vi "WFS Calc Spot To Reference Deviations.vi"(8 "error in (no error)":errorcluster {"code" format="%.0x"}, 10 "Cancel Wavefront Tilt (No)":i32(ring) items=["No", "Yes"], 11 "instrument handle":refnum<visa-resource-name>) -> (0 "error out":errorcluster {"code" format="%.0x"}, 3 "instrument handle out":refnum<visa-resource-name>)   [LabVIEW 2020]
doc: "This VI calculates reference positions and deviations for all spots depending on the setting ref_idx(internal/user) set by VI SetWavefrontReference.\nWhen option CancelWavefrontTilt is enabled the mean deviation in X and Y direction, which is measured within the pupil, is subtracted from the deviation data arrays.\n\nReference positions can be retrieved using VI GetSpotReferencePositions and calculated deviations by VI GetSpotDeviations."
uses:
  WFS_32.dll
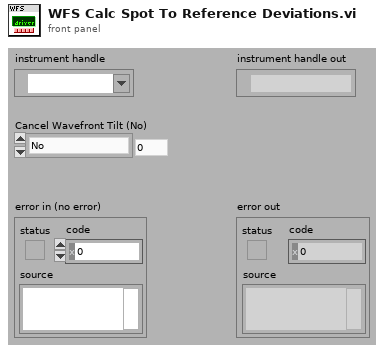
[diagram p1: front panel]
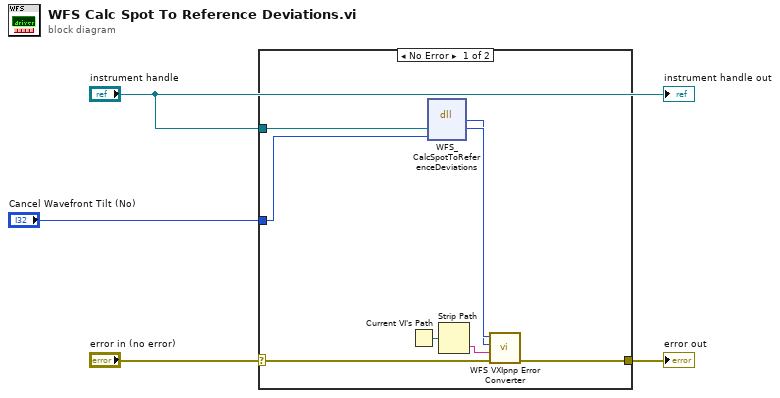
[diagram p0: block diagram]
diagram:
  n1 = case shown="No Error" "error in (no error)" {
    selector: "error in (no error)" -> [w7 w13]
    tunnel: [w6 w13] -> w4
    tunnel: "instrument handle" -> [w11 _]
    tunnel: "Cancel Wavefront Tilt (No)" -> [w5 _]
    frame No Error {
      n2 = Current VI's Path() -> (path=w12:path)
      n3 = dll-call lib="WFS_*.*" fn="WFS_CalcSpotToReferenceDeviations"("Instrument Handle"=w11, "Cancel Wavefront Tilt"=w5) -> (w9:i32, "Instrument Handle"=w10:u32)  [unwired: 4 in, 2 out]
      n4 = Strip Path(path=w12) -> (name=w8:string)  [unwired: 1 out]
      n5 = call "WFS VXIpnp Error Converter.vi"("error in (no error)"=w7, "Name Of VI (\"\")"=w8, "CVI Error Code (0)"=w9, "instrument handle"=w10) -> ("error out"=w6:errorcluster)  [unwired: 6 in, 1 out]
    }
    frame Error {
    }
  }
  "error out" <- w4
  "instrument handle out" <- "instrument handle"
